vi "publish.vi"(0 "HGF_DIMService":refnum<class "HGF_DIMService.lvclass">, 1 "typeDescriptor":string, 2 "data":variant, 3 "timeout in ms (-1)":i32, 5 "error in (no error)":errorcluster) -> (14 "dup HGF_DIMService":refnum<class "HGF_DIMService.lvclass">, 16 "rawData":variant, 17 "timed out?":bool, 19 "error out":errorcluster)   [LabVIEW 2012, in "HGF_DIM.lvlib" / "HGF_DIMService.lvclass"]
uses:
  HGF_DIMService.lvclass
  HGF_BaseClasses/HGF_PVPublisher/HGF_PVPublisher.lvclass
  HGF_DIMService.lvclass/HGF_DIMService.ctl
  DimLVEvent/LVDimInterface/LVDimInterface.lvlib
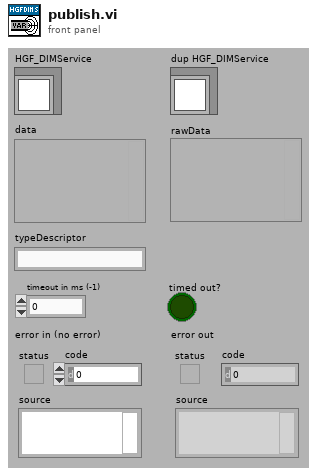
[diagram p1: front panel]
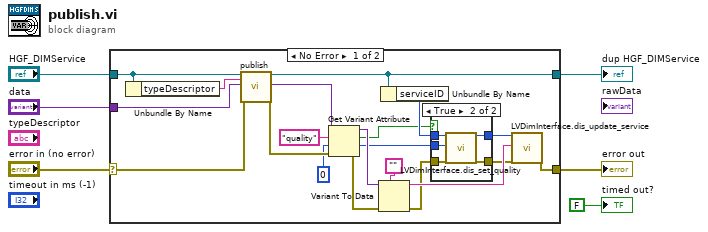
[diagram p0: block diagram]
diagram:
  n1 = case shown="No Error" "error in (no error)" {
    selector: "error in (no error)" -> [w8 w34]
    tunnel: "data" -> [w26 _]
    tunnel: [w24 w35] -> w5
    tunnel: [w10 w34] -> w4
    tunnel: "HGF_DIMService" -> [w9 w35]
    frame No Error {
      n2 = Unbundle By Name(w9) -> ("typeDescriptor"=w7:string)
      n3 = call-parent "publish.vi"("HGF_PVPublisher"=w9, "typeDescriptor"=w7, "data"=w26, "error in (no error)"=w8) -> ("dup HGF_PVPublisher"=w24:refnum<class "HGF_DIMService.lvclass">, "rawData"=w22:variant, "error out"=w20:errorcluster)  [unwired: 1 in, 12 out]
      n4 = Get Variant Attribute(Variant=w22, name="quality", default value (empty Variant)=0 ("quality"), error in=w20) -> (duplicate Variant=w21:variant, found=w11:bool, value=w12:i32, error out=w19:errorcluster)
      n5 = Variant To Data(error in=w19, type="", Variant=w21) -> (data=w23:string, error out=w14:errorcluster)
      n6 = Unbundle By Name(w24) -> ("serviceID"=w16:i32)
      n7 = case shown="True" w11 {
        tunnel: w16 -> [w28 w33]
        tunnel: [w28 w32] -> w15
        tunnel: w14 -> [w27 w31]
        tunnel: [w27 w30] -> w13
        tunnel: w12 -> [_ w29]
        frame False {
        }
        frame True {
          n8 = call "LVDimInterface.dis_set_quality.vi"("my_serviceID"=w33, "quality"=w29, "error in (no error)"=w31) -> ("my_serviceID (out)"=w32:i32, "error out"=w30:errorcluster)  [unwired: 15 out]
        }
      }
      n9 = call "LVDimInterface.dis_update_service.vi"("my_serviceID"=w15, "data"=w23, "error in (no error)"=w13) -> ("error out"=w10:errorcluster)  [unwired: 16 out]
    }
    frame Error {
    }
  }
  "error out" <- w4
  "dup HGF_DIMService" <- w5
  "timed out?" <- FALSE ("timed out?")
